vi "Plugin Config Parser.vi"(8 "error in":errorcluster, 11 "xml Path":path caption="path to XML document") -> (0 "error out":errorcluster, 3 "Custom Device Config out":refnum<data-value>)   [LabVIEW 2024, in "Config File Parser.lvlib"]
uses:
  Config File Parser.lvlib
  Custom Device Config/Custom Device Config.lvclass
  <vilib>/xml/Load XML File.vi
  <vilib>/xml/Close Reference(Node).vi
  <resource>/objmgr/DOMUserDefRef.rc
  <vilib>/xml/NI_XML.lvlib
panel:
  # "e"
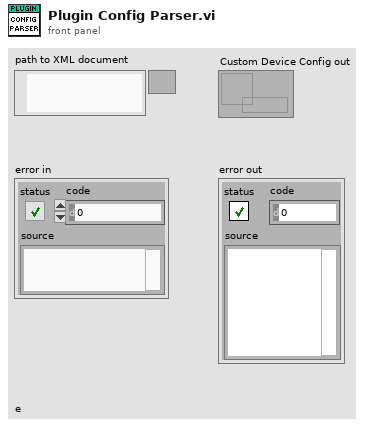
[diagram p1: front panel]
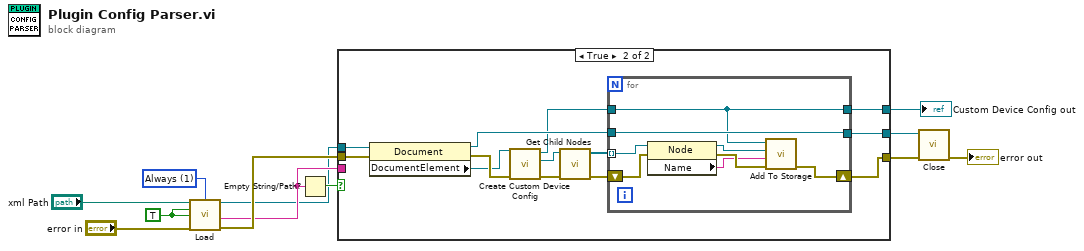
[diagram p0: block diagram]
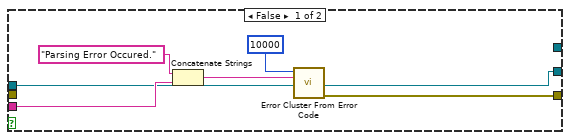
[diagram p2: hidden frame]
diagram:
  w5 = 1 items=["Never", "Always", "Auto"] ("Validate On Load")
  w6 = TRUE ("Do Namespaces")
  n1 = call-poly <vilib>:"Load.vi"("path to XML document"="xml Path", "validate on load (Auto)"=w5, "process namespaces (False)"=w6, "process schema (False)"=w6, "error in (no error)"="error in") -> ("DOM document out"=w2:refnum<k20>, "parse errors"=w3:string, "error out"=w9:errorcluster)  [unwired: 2 in, 6 out]
  n2 = Empty String/Path?(string/path=w3) -> (empty?=w7:bool)
  n3 = case shown="True" w7 {
    tunnel: w9 -> [_ w31]
    tunnel: w2 -> [w13 w26]
    tunnel: [w13 w24] -> w8
    tunnel: [w18 w27] -> w11
    tunnel: w3 -> [w16 _]
    tunnel: [_ w19] -> w1
    frame False {
      n4 = Concatenate Strings("Parsing Error Occured." ("error message (\"\")"), w16) -> (w14:string)
      n5 = call <vilib>:"Error Cluster From Error Code.vi"("error message (\"\")"=w14, "error code (0)"=10000) -> ("error out"=w18:errorcluster)  [unwired: 7 in]
    }
    frame True {
      n6 = property on="Property Node" class="Document"(reference=w26, error in=w31) -> (reference out=w23:refnum<k20>, error out=w29:errorcluster, "DocumentElement"=w22:refnum<k20>)
      n7 = call "Create Custom Device Config.vi"("error in"=w29, "XML Node"=w22) -> ("error out"=w28:errorcluster, "XML Node out"=w20:refnum<k20>, "Custom Device Config out"=w21:refnum<data-value>)  [unwired: 7 in]
      n8 = call "Get Child Nodes.vi"("error in"=w28, "Node"=w20) -> ("error out"=w30:errorcluster, "Child Nodes"=w25:refnum<k20>[])  [unwired: 8 in]
      n9 = for {
        tunnel: w25 -> [w36] mode=indexing
        tunnel: [w33] -> w24
        tunnel: w23 -> [w33]
        shift-right: [w37] -> w27
        shift-left: w30 -> [w39]
        tunnel: w21 -> [w32]
        tunnel: [w32] -> w19
        n10 = property on="Property Node" class="Node"(reference=w36, error in=w39) -> (reference out=w35:refnum<k20>, error out=w38:errorcluster, "Name"=w34:string)
        n11 = call "Add To Storage.vi"("error in"=w38, "Item Name"=w34, "Item node"=w35, "Item Ref in"=w32) -> ("error out"=w37:errorcluster)  [unwired: 6 in, 1 out]
      }
    }
  }
  "Custom Device Config out" <- w1
  n12 = call-poly <vilib>:"Close.vi"("error in (no error)"=w11, "node"=w8) -> ("error out"=→"error out":errorcluster)  [unwired: 7 in]
